vi "config_read.vi"(7 "name or relative path":string="config.ini", 8 "error in (no error)":errorcluster) -> (0 "error out":errorcluster, 3 "config data":T1)   [LabVIEW 2013]
uses:
  <vilib>/Utility/config.llb/Read Key (String).vi
  <vilib>/Utility/config.llb/Read Key (U32).vi
  <vilib>/Utility/config.llb/NI_LVConfig.lvlib
panel:
  in  "JSON_config_REST":T2
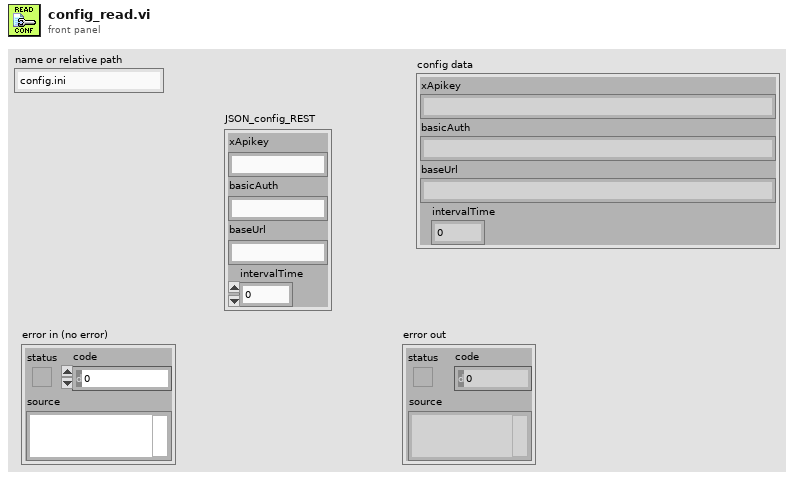
[diagram p1: front panel]
types:
  T1 = cluster{"xApikey":string, "basicAuth":string, "baseUrl":string, "intervalTime":i32}
  T2 = cluster{"xApikey":string, "basicAuth":string, "baseUrl":string, "intervalTime":u32}
  T3 = typedef "NI_LVConfig.lvlib/Config Data RefNum.ctl" = refnum<k1>
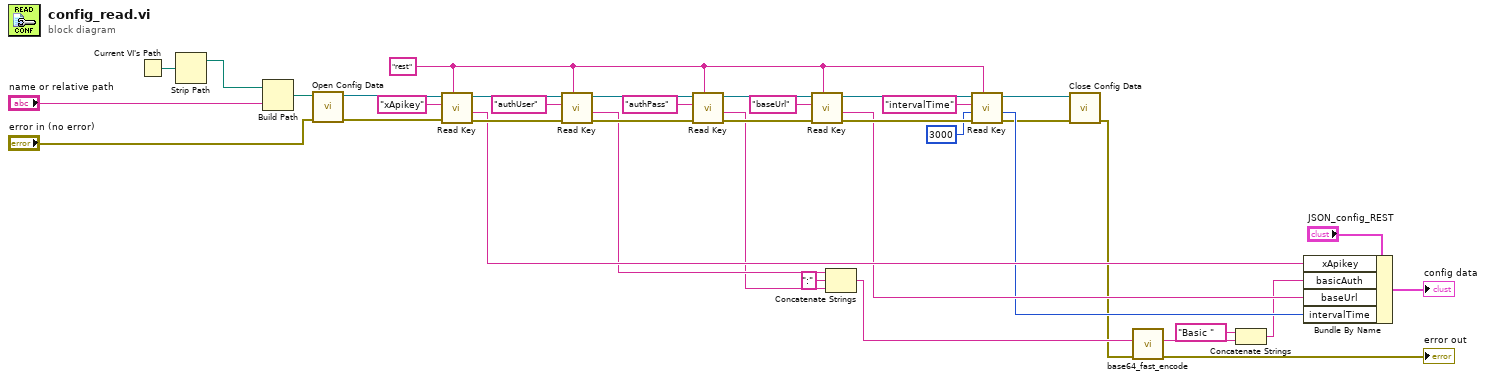
[diagram p0: block diagram]
diagram:
  w12 = "rest" ("section")
  n1 = Current VI's Path() -> (path=w38:path)
  n2 = Strip Path(path=w38) -> (stripped path=w37:path)  [unwired: 1 out]
  n3 = Build Path(base path=w37, name or relative path="name or relative path") -> (appended path=w8:path)
  n4 = call <vilib>:"Open Config Data.vi"("error in (no error)"="error in (no error)", "configuration file path"=w8) -> ("error out"=w25:errorcluster, "refnum"=w35:T3)  [unwired: 7 in, 1 out]
  n5 = call-poly <vilib>:"Read Key.vi"("section"=w12, "error in (no error)"=w25, "key"="xApikey", "refnum"=w35) -> ("error out"=w24:errorcluster, "value"=w19:string, "refnum out"=w29:T3)  [unwired: 4 in, 1 out]
  n6 = call-poly <vilib>:"Read Key.vi"("section"=w12, "error in (no error)"=w24, "key"="authUser", "refnum"=w29) -> ("error out"=w23:errorcluster, "value"=w18:string, "refnum out"=w28:T3)  [unwired: 4 in, 1 out]
  n7 = call-poly <vilib>:"Read Key.vi"("section"=w12, "error in (no error)"=w23, "key"="authPass", "refnum"=w28) -> ("error out"=w22:errorcluster, "value"=w16:string, "refnum out"=w27:T3)  [unwired: 4 in, 1 out]
  n8 = call-poly <vilib>:"Read Key.vi"("section"=w12, "error in (no error)"=w22, "key"="baseUrl", "refnum"=w27) -> ("error out"=w21:errorcluster, "value"=w15:string, "refnum out"=w26:T3)  [unwired: 4 in, 1 out]
  n9 = Concatenate Strings(w18, ":" ("string"), w16) -> (w5:string)
  n10 = call-poly <vilib>:"Read Key.vi"("section"=w12, "error in (no error)"=w21, "default value"=u32 3000, "key"="intervalTime", "refnum"=w26) -> ("error out"=w10:errorcluster, "value"=w14:u32, "refnum out"=w9:T3)  [unwired: 3 in, 1 out]
  n11 = call <vilib>:"Close Config Data.vi"("error in (no error)"=w10, "refnum"=w9) -> ("error out"=w3:errorcluster)  [unwired: 8 in, 1 out]
  n12 = call "base64_fast_encode.vi"("error in (no error)"=w3, "string in (not encoded)"=w5) -> ("error out"=→"error out":errorcluster, "string out (base64-encoded)"=w7:string)  [unwired: 8 in]
  n13 = Concatenate Strings("Basic " ("string"), w7) -> (w4:string)
  n14 = Bundle By Name(cluster="JSON_config_REST", "xApikey"=w19, "basicAuth"=w4, "baseUrl"=w15, "intervalTime"=w14) -> (→"config data":T2)
